vi "Create Definition.vi"(9 "Header":refnum<class "Linked List Header.lvclass">, 10 "Unique ID":string, 11 "Name":string) -> (3 "Linked List Definition out":refnum<class "Linked List Definition.lvclass">)   [LabVIEW 2020, in "Linked Lists.lvlib" / "Linked List Definition.lvclass"]
uses:
  <vilib>/gpm_packages/@cs/linked-list/Source/Linked List/Linked List Definition/Linked List Definition.lvclass
  <vilib>/gpm_packages/@cs/linked-list/Source/Linked List/Linked List Header/Linked List Header.lvclass
  <vilib>/gpm_packages/@cs/linked-list/Source/Linked List/Linked List Definition/Linked List Definition.lvclass/Linked List Definition.ctl
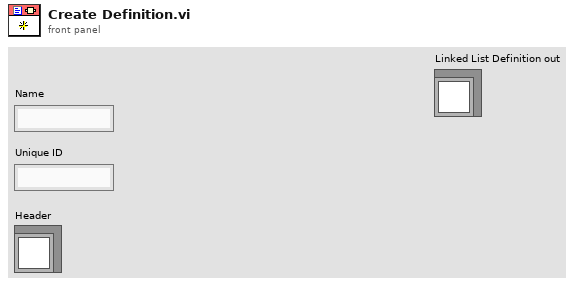
[diagram p1: front panel]
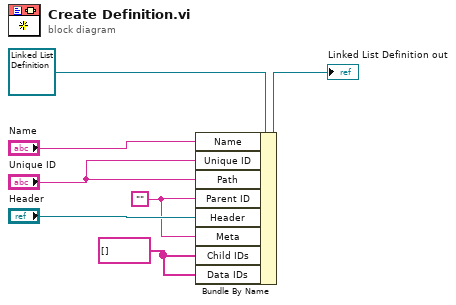
[diagram p0: block diagram]
diagram:
  w1 = string[] [] ("Child IDs")
  w2 = ""
  n1 = Bundle By Name(cluster=refnum<class "Linked List Definition.lvclass"> refnum ("Linked List Definition in"), "Name"="Name", "Unique ID"="Unique ID", "Path"="Unique ID", "Parent ID"=w2, "Header"="Header", "Meta"=w2, "Child IDs"=w1, "Data IDs"=w1) -> (→"Linked List Definition out":refnum<class "Linked List Definition.lvclass">)
